vi "test-linear-system-loop-01.vi"() -> (3 "TEst Passed":bool)   [LabVIEW 2019]
uses:
  <vilib>/Rock Robotics/WPI/ThirdParty/JAS_Junk/TrajLib/LINEAR_SYSTEM_LOOP.ctl
  <vilib>/Rock Robotics/WPI/ThirdParty/JAS_Junk/TrajLib/LINEAR_QUADRATIC_REGULATOR.ctl
  <vilib>/Analysis/Matrix/Datatypes/RealMatrix.ctl
  <vilib>/Rock Robotics/WPI/ThirdParty/JAS_Junk/TrajLib/LINEAR_PLANT_INV_FF.ctl
  <vilib>/Rock Robotics/WPI/ThirdParty/JAS_Junk/TrajLib/KALMAN_FILTER.ctl
  <vilib>/Rock Robotics/WPI/ThirdParty/JAS_Junk/TrajLib/LINEAR_SYSTEM.ctl
  <vilib>/Rock Robotics/WPI/ThirdParty/JAS_Junk/TrajLib/DCMOTOR_TYPES_ENUM.ctl
  <vilib>/Rock Robotics/WPI/ThirdParty/JAS_Junk/TrajLib/MatBuilder_Create.vi
  <vilib>/Rock Robotics/WPI/ThirdParty/JAS_Junk/TrajLib/DCMotor_GetCIM.vi
  <vilib>/Rock Robotics/WPI/ThirdParty/JAS_Junk/TrajLib/DCMotor_GetAndymark9015.vi
  <vilib>/Rock Robotics/WPI/ThirdParty/JAS_Junk/TrajLib/DCMotor_GetAndymarkRs775_125.vi
  <vilib>/Rock Robotics/WPI/ThirdParty/JAS_Junk/TrajLib/DCMotor_GetBag.vi
  <vilib>/Rock Robotics/WPI/ThirdParty/JAS_Junk/TrajLib/DCMotor_GetBanebotsRs550.vi
  <vilib>/Rock Robotics/WPI/ThirdParty/JAS_Junk/TrajLib/DCMotor_GetBanebotsRs775.vi
  <vilib>/Rock Robotics/WPI/ThirdParty/JAS_Junk/TrajLib/DCMotor_GetFalcon500.vi
  <vilib>/Rock Robotics/WPI/ThirdParty/JAS_Junk/TrajLib/DCMotor_GetMiniCIM.vi
  <vilib>/Rock Robotics/WPI/ThirdParty/JAS_Junk/TrajLib/DCMotor_GetNEO.vi
  <vilib>/Rock Robotics/WPI/ThirdParty/JAS_Junk/TrajLib/DCMotor_GetNEO550.vi
  <vilib>/Rock Robotics/WPI/ThirdParty/JAS_Junk/TrajLib/DCMotor_GetRomiBuiltIn.vi
  <vilib>/Rock Robotics/WPI/ThirdParty/JAS_Junk/TrajLib/DCMotor_GetVex775Pro.vi
  <vilib>/Rock Robotics/WPI/ThirdParty/JAS_Junk/TrajLib/LinearSystem_New.vi
  <vilib>/Rock Robotics/WPI/ThirdParty/JAS_Junk/TrajLib/MatBuilder_Fill.vi
  <vilib>/Rock Robotics/WPI/ThirdParty/JAS_Junk/TrajLib/MatrixHelper_Zero.vi
  <vilib>/Rock Robotics/WPI/ThirdParty/JAS_Junk/TrajLib/TrapProfile_ShouldFlipAcceleration.vi
  <vilib>/Rock Robotics/WPI/ThirdParty/JAS_Junk/TrajLib/TrapProfile_Direct.vi
  <vilib>/Rock Robotics/SystemInterfaces/NetworkCommunication/NetComm_UsageReport_report.vi
  <vilib>/Rock Robotics/WPI/ThirdParty/JAS_Junk/TrajLib/DCMotor_New.vi
  <vilib>/Rock Robotics/WPI/ThirdParty/JAS_Junk/TrajLib/Units_RotationsPerMinuteToRadiansPerSecond.vi
  <vilib>/Rock Robotics/WPI/ThirdParty/JAS_Junk/TrajLib/MatrixHelper_CoerceSize.vi
  <vilib>/Rock Robotics/WPI/ThirdParty/JAS_Junk/TrajLib/Util_LibraryGlobals.vi
  <vilib>/Rock Robotics/WPI/ThirdParty/JAS_Junk/TrajLib/Trajectory_Library.lvlib
  <vilib>/ptbypt/NI_PtbyPt.lvlib
  <vilib>/Analysis/Matrix/NI_Matrix.lvlib
panel:
  out "Waveform Graph":dbl[][](graph)
  out "Issue":bool
  out "Error":bool
  out "CorrError":bool
  out "out Linear System Loop":T1
  out "CalcYErr":bool
  out "LinSysLoopErr":bool
  out "LQRError":bool
  out "KalmanError":bool
  out "Elev Sstem Err":bool
  # "<States,1>"
  # "<FUTURE --- CLAMP TYPE -- For now\nuse Normalize>"
  # "Steady State Gain  \n<States,Outputs>"
  # "State Estimate <Statess,1>"
  # "<States,States>"
  # "<States,Inputs>"
  # "<Outputs,States>"
  # "<Outputs,Inputs>"
  # "<States,1>"
  # "<Inputs,1>"
  # "<States,Inputs>"
  # "<States,States>"
  # "Ref State <States,1>"
  # "Comp and capped \noutput <Inputs,1>"
  # "Controller gain\n<Inputs,States>"
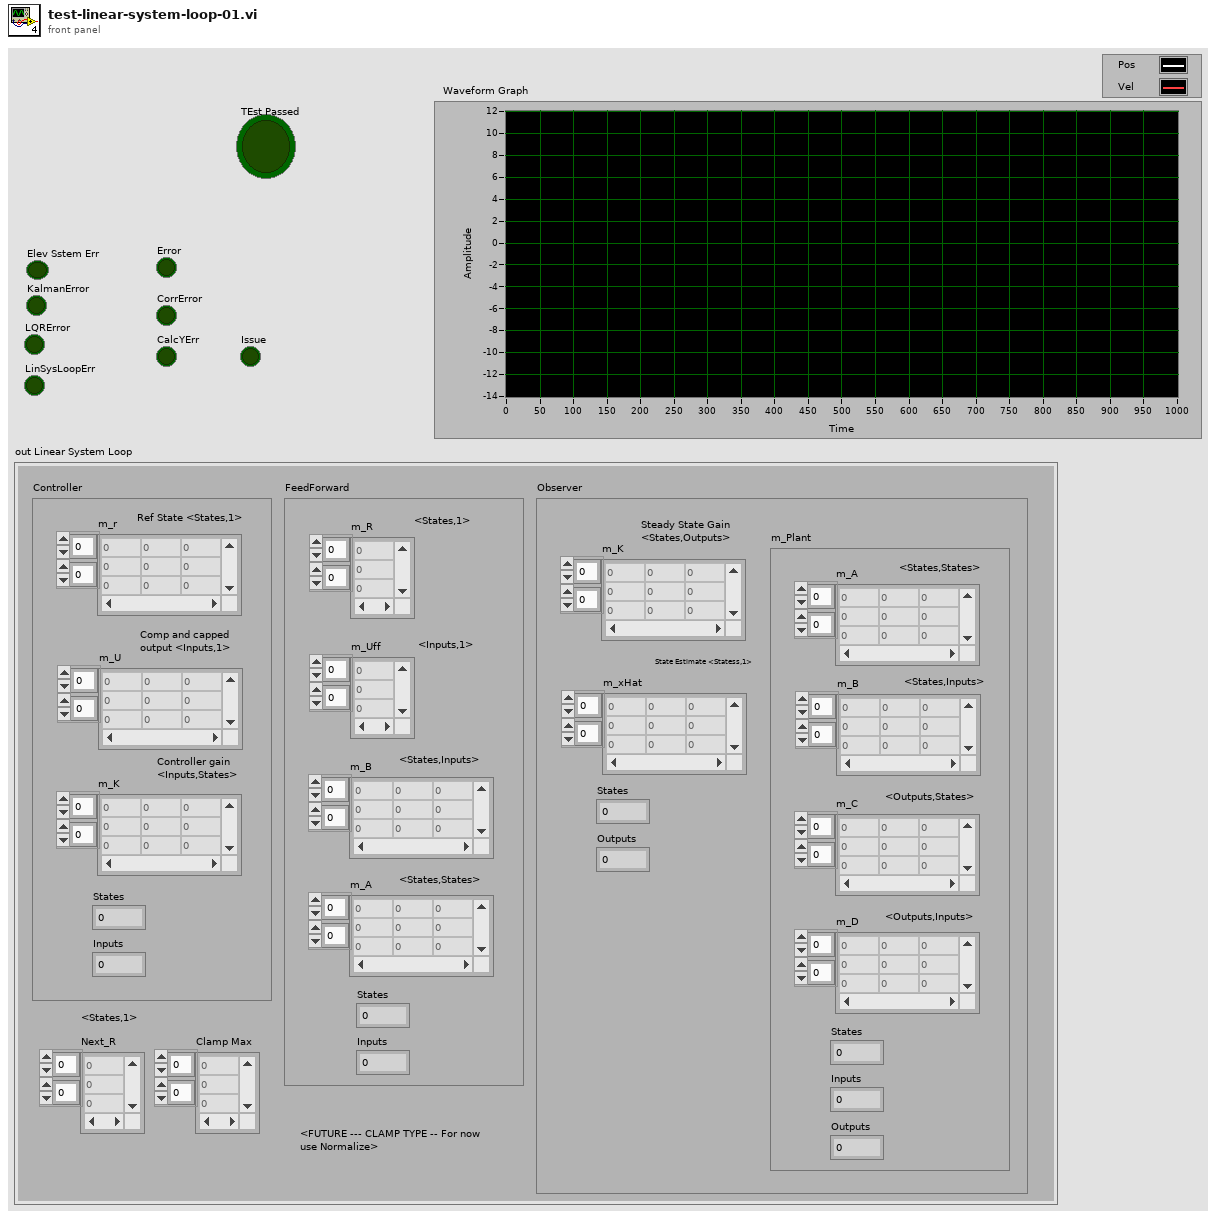
[diagram p1: front panel]
types:
  T1 = typedef "Trajectory_Library.lvlib/LINEAR_SYSTEM_LOOP.ctl" = cluster{"Controller":T2, "FeedForward":T4, "Observer":T5, "Next_R":T3, "Clamp Max":T3}
  T2 = typedef "Trajectory_Library.lvlib/LINEAR_QUADRATIC_REGULATOR.ctl" = cluster{"m_r":T3, "m_U":T3, "m_K":T3, "States":i32, "Inputs":i32}
  T3 = typedef "NI_Matrix.lvlib/RealMatrix.ctl" = dbl[][]
  T4 = typedef "Trajectory_Library.lvlib/LINEAR_PLANT_INV_FF.ctl" = cluster{"m_R":T3, "m_Uff":T3, "m_B":T3, "m_A":T3, "States":i32, "Inputs":i32}
  T5 = typedef "Trajectory_Library.lvlib/KALMAN_FILTER.ctl" = cluster{"m_K":T3, "m_xHat":T3, "States":i32, "Outputs":i32, "m_Plant":T6}
  T6 = typedef "Trajectory_Library.lvlib/LINEAR_SYSTEM.ctl" = cluster{"m_A":T3, "m_B":T3, "m_C":T3, "m_D":T3, "States":i32, "Inputs":i32, "Outputs":i32}
  T7 = typedef "Trajectory_Library.lvlib/DCMOTOR_TYPES_ENUM.ctl" = enum16{"CIM", "AndyMark 9015", "Andy Mark RS 775 125", "Bag", "BaneBots RS 550", "BaneBots RS 775", "Falcon 500", "Mini CIM", "NEO", "NEO 550", "Romi BuiltIn", "Vex 775 Pro"}
  T8 = typedef "Trajectory_Library.lvlib/DCMOTOR.CTL" = cluster{"nominalVoltage_Volts":dbl, "StallTorque_NM":dbl, "StallCurrent_Amps":dbl, "FreeCurrent_Amps":dbl, "FreeSpeed_RadPerSec":dbl, "R_Ohms":dbl, "KvINV_RadPerSecPerVolt":dbl, "Kt_NMPerAmp":dbl, "L_H":dbl, "Jr_KgM2":dbl}
  T9 = typedef "Trajectory_Library.lvlib/TRAPEZOID_PROFILE_CONSTRAINT.ctl" = cluster{"MaxVelocity":dbl, "MaxAcceleration":dbl}
  T10 = typedef "Trajectory_Library.lvlib/TRAPEZOID_PROFILE_STATE.ctl" = cluster{"Position":dbl, "Velocity":dbl}
  T11 = typedef "Trajectory_Library.lvlib/TRAPEZOID_PROFILE.ctl" = cluster{"EndAccel":dbl, "EndFullSpeed":dbl, "EndDecel":dbl, "Direction":i32, "Constraints":T9, "Initial":T10, "Goal":T10}
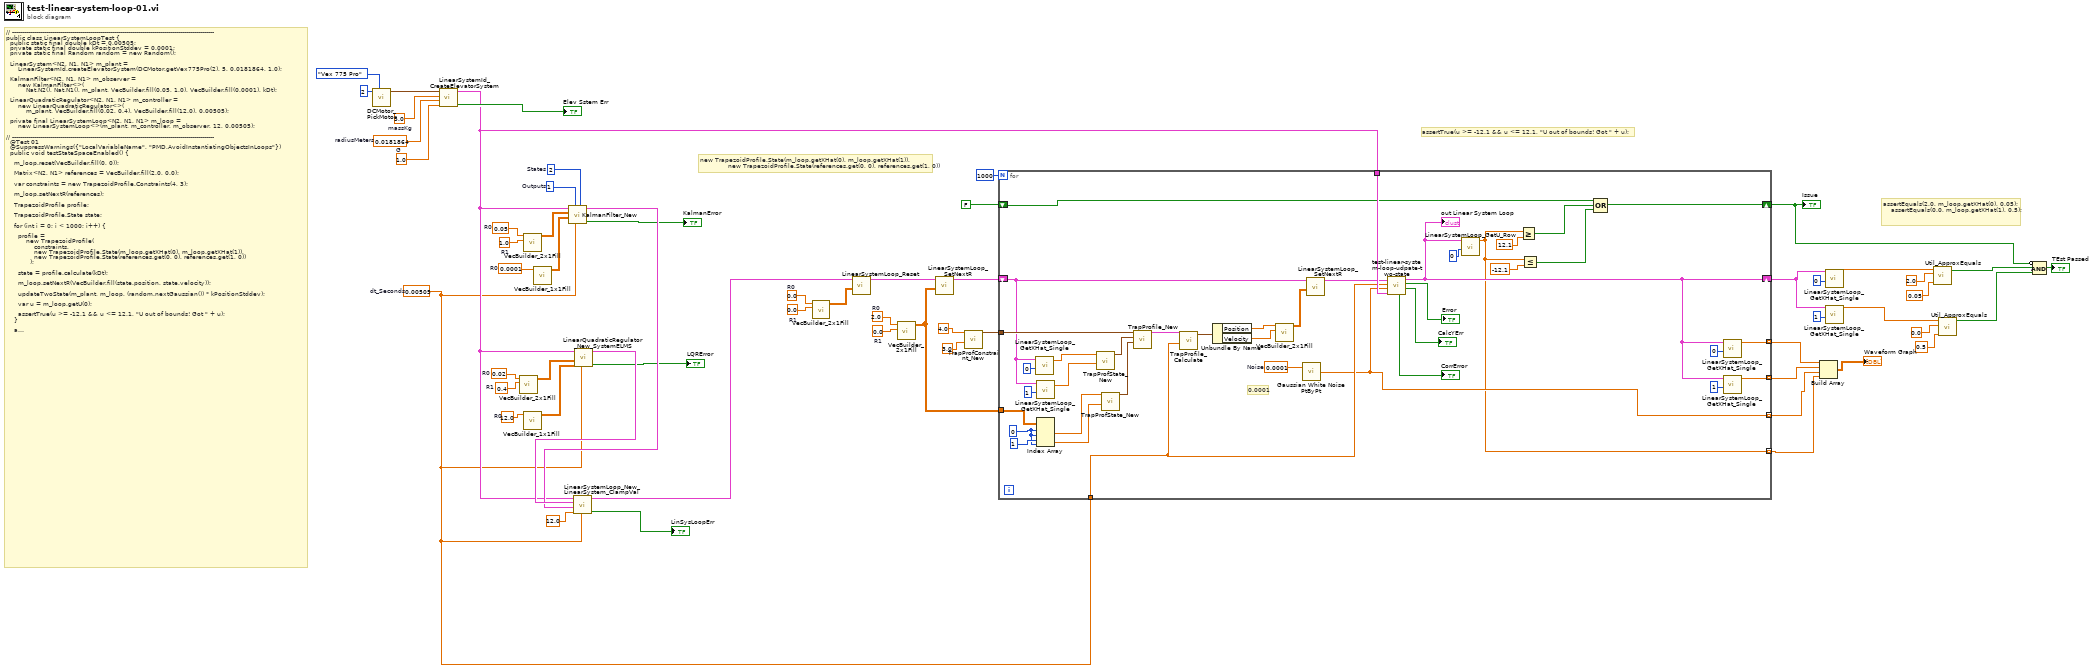
[diagram p0: block diagram]
diagram:
  w28 = 0.0  # R1
  w27 = 2.0  # R0
  w35 = 0.0  # R1
  w34 = 0.0  # R0
  w45 = 12.0  # R0
  w47 = 0.4  # R1
  w46 = 0.02  # R0
  w49 = 0.0001  # R0
  w51 = 1.0  # R1
  w50 = 0.05  # R0
  w52 = 1  # Outputs
  w21 = 0.00505  # dt_Seconds
  w53 = 2  # States
  w57 = 5.0  # massKg
  w58 = 0.0181864  # radiusMeters
  w59 = 1.0  # G
  # "assertEquals(2.0, m_loop.getXHat(0), 0.05);\n    assertEquals(0.0, m_loop.getXHat(1), 0.5);"
  # "assertTrue(u >= -12.1 && u <= 12.1, \"U out of bounds! Got \" + u);"
  # "new TrapezoidProfile.State(m_loop.getXHat(0), m_loop.getXHat(1)),\n              new TrapezoidProfile.State(references.get(0, 0), references.get(1, 0))"
  # "// -----------------------------------------------------------------------------------------------------\npublic class LinearSystemLoopTest {\n  public static final double kDt = 0.00505;\n  private static final double kPositionStddev = 0.0001;\n  private static final Random random = new Random();\n\n  LinearSystem<N2, N1, N1> m_plant =\n      LinearSystemId.createElevatorSystem(DCMotor.getVex775Pro(2), 5, 0.0181864, 1.0);\n\n  KalmanFilter<N2, N1, N1> m_observer =\n      new KalmanFilter<>(\n          Nat.N2(), Nat.N1(), m_plant, VecBuilder.fill(0.05, 1.0), VecBuilder.fill(0.0001), kDt);\n\n  LinearQuadraticRegulator<N2, N1, N1> m_controller =\n      new LinearQuadraticRegulator<>(\n          m_plant, VecBuilder.fill(0.02, 0.4), VecBuilder.fill(12.0), 0.00505);\n\n  private final LinearSystemLoop<N2, N1, N1> m_loop =\n      new LinearSystemLoop<>(m_plant, m_controller, m_observer, 12, 0.00505);\n\n// -----------------------------------------------------------------------------------------------------\n  @Test 01\n  @SuppressWarnings({\"LocalVariableName\", \"PMD.AvoidInstantiatingObjectsInLoops\"})\n  public void testStateSpaceEnabled() {\n\n    m_loop.reset(VecBuilder.fill(0, 0));\n\n    Matrix<N2, N1> references = VecBuilder.fill(2.0, 0.0);\n\n    var constraints = new TrapezoidProfile.Constraints(4, 3);\n\n    m_loop.setNextR(references);\n\n    TrapezoidProfile profile;\n\n    TrapezoidProfile.State state;\n\n    for (int i = 0; i < 1000; i++) {\n\n      profile =\n          new TrapezoidProfile(\n              constraints,\n              new TrapezoidProfile.State(m_loop.getXHat(0), m_loop.getXHat(1)),\n              new TrapezoidProfile.State(references.get(0, 0), references.get(1, 0))\n            );\n\n      state = profile.calculate(kDt);\n\n      m_loop.setNextR(VecBuilder.fill(state.position, state.velocity));\n\n      updateTwoState(m_plant, m_loop, (random.nextGaussian()) * kPositionStddev);\n\n      var u = m_loop.getU(0);\n\n      assertTrue(u >= -12.1 && u <= 12.1, \"U out of bounds! Got \" + u);\n    }\n\n    assertEquals(2.0, m_loop.getXHat(0), 0.05);\n    assertEquals(0.0, m_loop.getXHat(1), 0.5);\n  }"
  n1 = call <vilib>:"DCMotor_PickMotor.vi"("DCMOTOR_TYPES"=DCMOTOR_TYPES_ENUM."Vex 775 Pro", "Num Motors"=2) -> ("DCMOTOR"=w54:T8)  [unwired: 9 in]
  n2 = call <vilib>:"LinearSystemId_CreateElevatorSystem.vi"("G"=w59, "radiusMeters"=w58, "massKg"=w57, "DCMOTOR"=w54) -> ("Size Coerced"=→"Elev Sstem Err":bool, "Linearsystem"=w33:T6)  [unwired: 6 in]
  n3 = call <vilib>:"VecBuilder_2x1Fill.vi"("R1"=w47, "R0"=w46) -> ("output matrix"=w44:T3)  [unwired: 9 in]
  n4 = call <vilib>:"VecBuilder_1x1Fill.vi"("R0_C0"=w45) -> ("output matrix"=w43:T3)  [unwired: 10 in]
  n5 = call <vilib>:"VecBuilder_2x1Fill.vi"("R1"=w51, "R0"=w50) -> ("output matrix"=w48:T3)  [unwired: 9 in]
  n6 = call <vilib>:"VecBuilder_1x1Fill.vi"("R0_C0"=w49) -> ("output matrix"=w26:T3)  [unwired: 10 in]
  n7 = call <vilib>:"KalmanFilter_New.vi"("States"=w53, "dt_Seconds"=w21, "Outputs"=w52, "MeasurementStdDevs"=w26, "StateStdDevs"=w48, "Plant"=w33) -> ("Error"=→"KalmanError":bool, "KalmanFilter"=w41:T5)  [unwired: 4 in]
  n8 = call <vilib>:"LinearQuadraticRegulator_New_SystemELMS.vi"("dt_Seconds"=w21, "Relms"=w43, "Qelms"=w44, "LINEARSYSTEM"=w33) -> ("Error"=→"LQRError":bool, "LinearQuadraticRegulator"=w42:T2)  [unwired: 6 in]
  n9 = call <vilib>:"LinearSystemLoop_New_LinearSystem_ClampVal.vi"("dT_Seconds"=w21, "Max_Voltage"=12.0, "Observer"=w41, "Controller"=w42, "Plant"=w33) -> ("Error"=→"LinSysLoopErr":bool, "Linear System Loop"=w32:T1)  [unwired: 5 in]
  n10 = call <vilib>:"VecBuilder_2x1Fill.vi"("R1"=w35, "R0"=w34) -> ("output matrix"=w31:T3)  [unwired: 9 in]
  n11 = call <vilib>:"LinearSystemLoop_Reset.vi"("initialState"=w31, "input inear System Loop"=w32) -> ("out Linear System Loop"=w30:T1)  [unwired: 8 in, 1 out]
  n12 = call <vilib>:"VecBuilder_2x1Fill.vi"("R1"=w28, "R0"=w27) -> ("output matrix"=w20:T3)  [unwired: 9 in]
  n13 = call <vilib>:"LinearSystemLoop_SetNextR.vi"("R"=w20, "input inear System Loop"=w30) -> ("out Linear System Loop"=w29:T1)  [unwired: 8 in, 1 out]
  n14 = call <vilib>:"TrapProfConstraint_New.vi"("Max Accel"=3.0, "Max Speed (M/S)"=4.0) -> ("TRAPEZOID_PROFILE_CONSTRAINT"=w22:T9)  [unwired: 9 in]
  n15 = for {
    N: 1000 -> [_]
    tunnel: w33 -> [w95]
    tunnel: w21 -> [w81]
    shift-right: [w64] -> w18
    shift-left: w29 -> [w77]
    tunnel: w22 -> [w94]
    tunnel: w20 -> [w85]
    shift-right: [w68] -> w6
    shift-left: FALSE -> [w67]
    tunnel: [w63] -> w9 mode=indexing
    tunnel: [w62] -> w8 mode=indexing
    tunnel: [w61] -> w2 mode=indexing
    tunnel: [w60] -> w1 mode=indexing
    w86 = 0 ("index (row)")
    w74 = 0.0001  # Noise
    # "0.0001"
    n16 = call <vilib>:"LinearSystemLoop_GetXHat_Single.vi"("Row"=0, "input inear System Loop"=w77) -> ("XHat"=w89:dbl)  [unwired: 9 in]
    n17 = call <vilib>:"LinearSystemLoop_GetXHat_Single.vi"("Row"=1, "input inear System Loop"=w77) -> ("XHat"=w88:dbl)  [unwired: 9 in]
    n18 = Index Array(array=w85, index (row) #1=w86, index (col) #1=w86, index (row) #2=1 ("index (row)"), index (col) #2=w86) -> (element #1=w84:dbl, element #2=w83:dbl)
    n19 = call <vilib>:"TrapProfState_New.vi"("Velocity"=w88, "Position"=w89) -> ("TRAPEZOID_PROFILE_STATE"=w93:T10)  [unwired: 9 in]
    n20 = call <vilib>:"TrapProfState_New.vi"("Velocity"=w83, "Position"=w84) -> ("TRAPEZOID_PROFILE_STATE"=w92:T10)  [unwired: 9 in]
    n21 = call <vilib>:"TrapProfile_New.vi"("Initial"=w92, "Goal"=w93, "Constraints"=w94) -> ("TRAPEZOID_PROFILE"=w82:T11)  [unwired: 8 in]
    n22 = call <vilib>:"TrapProfile_Calculate.vi"("Time"=w81, "TRAPEZOID_PROFILE"=w82) -> ("State"=w80:T10)  [unwired: 9 in]
    n23 = Unbundle By Name(w80) -> ("Position"=w79:dbl, "Velocity"=w78:dbl)
    n24 = call <vilib>:"VecBuilder_2x1Fill.vi"("R1"=w78, "R0"=w79) -> ("output matrix"=w75:T3)  [unwired: 9 in]
    n25 = call <vilib>:"Gaussian White Noise PtByPt.vi"("standard deviation"=w74) -> ("Gaussian white noise"=w61:dbl)  [unwired: 2 in]
    n26 = call <vilib>:"LinearSystemLoop_SetNextR.vi"("R"=w75, "input inear System Loop"=w77) -> ("out Linear System Loop"=w76:T1)  [unwired: 8 in, 1 out]
    n27 = call "test-linear-system-loop-udpate-two-state.vi"("Linearsystem"=w95, "Noise"=w61, "dt_Seconds"=w81, "Linear System Loop"=w76) -> ("CalcYErr"=→"CalcYErr":bool, "PredictError"=→"Error":bool, "out Linear System Loop"=w64:T1, "CorrectError"=→"CorrError":bool)  [unwired: 4 in]
    "out Linear System Loop" <- w64
    n28 = call <vilib>:"LinearSystemLoop_GetU_Row.vi"("Row"=0, "input inear System Loop"=w64) -> ("U"=w60:dbl)  [unwired: 9 in]
    n29 = Greater Or Equal?(x=w60, y=12.1) -> (x >= y?=w69:bool)
    n30 = Less Or Equal?(x=w60, y=-12.1) -> (x <= y?=w70:bool)
    n31 = Compound Arithmetic op=OR(w67, w69, w70) -> (w68:bool)
    n32 = call <vilib>:"LinearSystemLoop_GetXHat_Single.vi"("Row"=0, "input inear System Loop"=w64) -> ("XHat"=w63:dbl)  [unwired: 9 in]
    n33 = call <vilib>:"LinearSystemLoop_GetXHat_Single.vi"("Row"=1, "input inear System Loop"=w64) -> ("XHat"=w62:dbl)  [unwired: 9 in]
  }
  "Issue" <- w6
  n34 = Build Array(w9, w8, w2, w1) -> (→"Waveform Graph":dbl[][])
  n35 = call <vilib>:"LinearSystemLoop_GetXHat_Single.vi"("Row"=0, "input inear System Loop"=w18) -> ("XHat"=w13:dbl)  [unwired: 9 in]
  n36 = call <vilib>:"LinearSystemLoop_GetXHat_Single.vi"("Row"=1, "input inear System Loop"=w18) -> ("XHat"=w10:dbl)  [unwired: 9 in]
  n37 = call <vilib>:"Util_ApproxEquals.vi"("Tolerance"=0.05, "Value 2"=2.0, "Value 1"=w13) -> ("ApproxEquals"=w5:bool)  [unwired: 8 in]
  n38 = call <vilib>:"Util_ApproxEquals.vi"("Tolerance"=0.5, "Value 2"=0.0, "Value 1"=w10) -> ("ApproxEquals"=w4:bool)  [unwired: 8 in]
  n39 = Compound Arithmetic op=AND(invert w6, w5, w4) -> (→"TEst Passed":bool)
